vi "VIS-IR_Stop_ring.vi"(8 "error in (no error)":errorcluster, 11 "VIS-IR in":refnum<class "VIS-NIR.lvclass">) -> (0 "error out":errorcluster, 3 "VIS-IR out":refnum<class "VIS-NIR.lvclass">)   [LabVIEW 2018, in "VIS-NIR.lvclass"]
uses:
  VIS-NIR.lvclass
  C:/Users/Sergey Denisov/Documents/REPS/TRANCON/Classes/Detector/Detector.lvclass
  Detector.lvclass/Detector.ctl
  Detector.lvclass
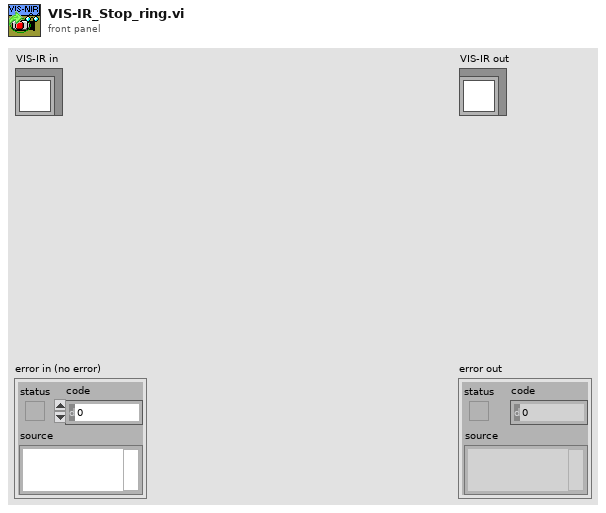
[diagram p1: front panel]
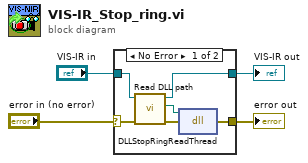
[diagram p0: block diagram]
diagram:
  n1 = case shown="No Error" "error in (no error)" {
    selector: "error in (no error)" -> [w9 w12]
    tunnel: [w6 w12] -> w3
    tunnel: [w5 w11] -> w1
    tunnel: "VIS-IR in" -> [w10 w11]
    frame No Error {
      n2 = call "Read DLL path.vi"("error in (no error)"=w9, "Detector in"=w10) -> ("error out"=w7:errorcluster, "DLL path"=w8:path, "Detector out"=w5:refnum<class "VIS-NIR.lvclass">)  [unwired: 7 in]
      n3 = dll-call lib="G:/SD/TRANCON/DLL/ESLSCDLL.dll" fn="DLLStopRingReadThread"(path in=w8, error in=w7) -> (error out=w6:errorcluster)  [unwired: 2 in, 1 out]
    }
    frame Error {
    }
  }
  "error out" <- w3
  "VIS-IR out" <- w1
